vi "User Command Registers.vi"(0 "register instruction":T2) -> (4 "read completion":T1, 8 "IO Module\\User Command Idle":bool, 10 "IO Module\\User Error":u8, 14 "ready for input":bool)   [LabVIEW 2013]
uses:
  <instrlib>/ni579x/Register Bus/v1/FPGA/Public/Register Instruction.ctl
  <instrlib>/ni579x/Register Bus/v1/FPGA/Public/Read Completion.ctl
  <instrlib>/ni579x/Config/v1/Shared/Types/ni579x Register Bus Subsystem ID.ctl
  <vilib>/rvi/eio/common/nirviEmuTemplateMethod_errors.vi
  <vilib>/eio/EIONode/EIONode.xnode
  <vilib>/rvi/DataTransferAndStorage/Container/XNode/niFpgaContainer.xnode
  <instrlib>/ni579x/Register Bus/v1/FPGA/ni579x Register Bus v1 FPGA.lvlib
  <vilib>/rvi/interface/RandomDataEmulation/nirviRandomDataFpgaReadWriteTemplate.vi
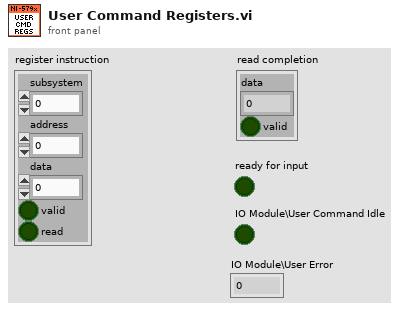
[diagram p1: front panel]
types:
  T1 = typedef "ni579x Register Bus v1 FPGA.lvlib/Read Completion.ctl" = cluster{"data":u32, "valid":bool}
  T2 = typedef "ni579x Register Bus v1 FPGA.lvlib/Register Instruction.ctl" = cluster{"subsystem":u8, "address":u16, "data":u32, "valid":bool, "read":bool}
  T3 = typedef "ni579x Register Bus Subsystem ID.ctl" = u8
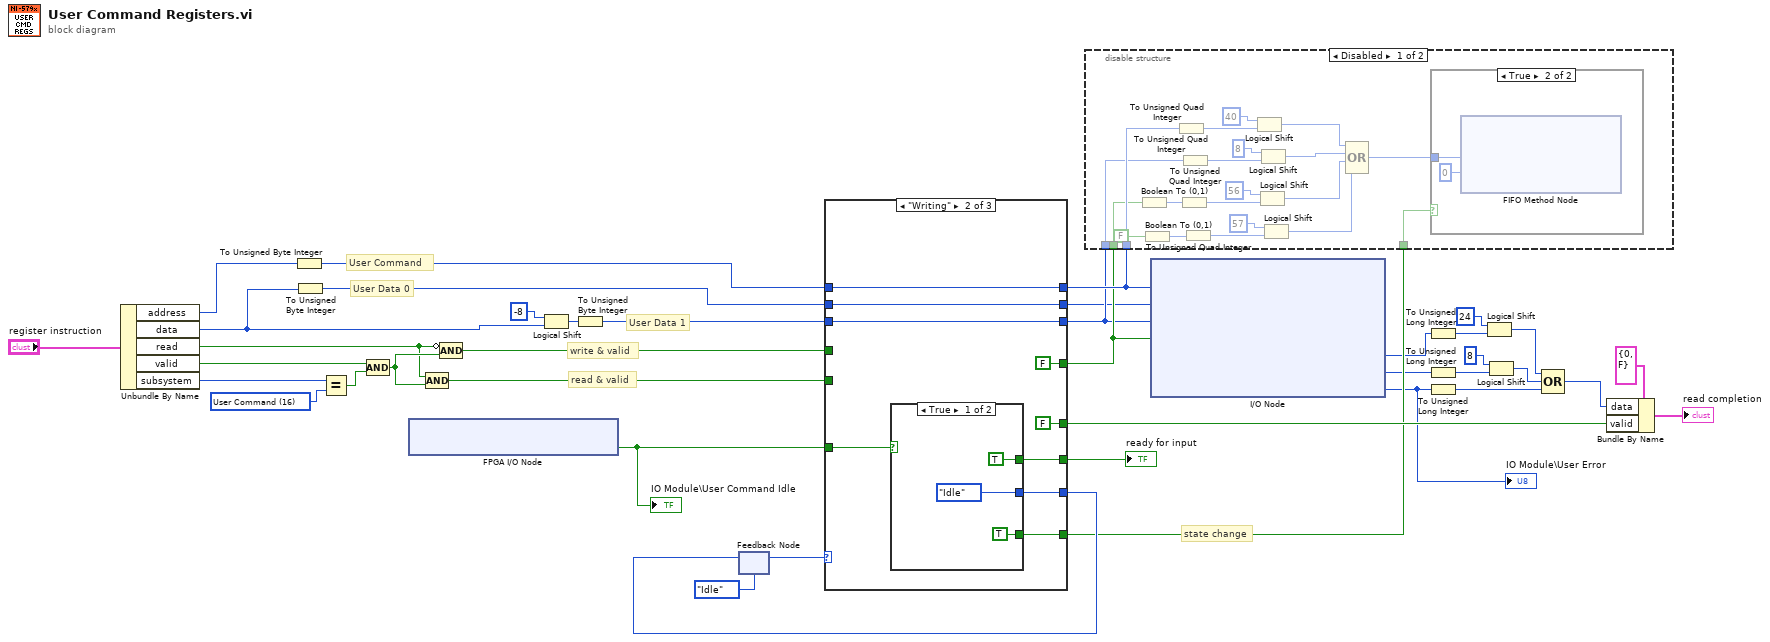
[diagram p0: block diagram]
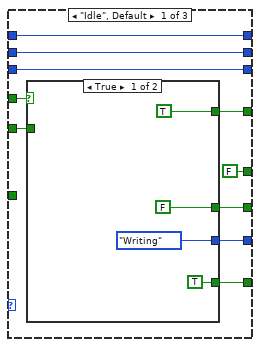
[diagram p4: hidden frame]
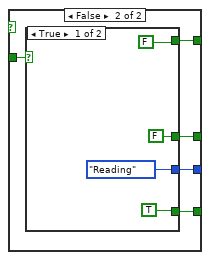
[diagram p5: hidden frame]
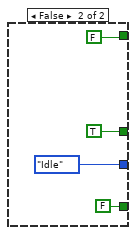
[diagram p6: hidden frame]
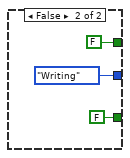
[diagram p7: hidden frame]
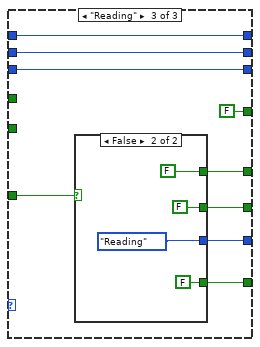
[diagram p8: hidden frame]
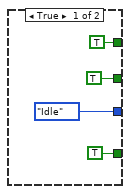
[diagram p9: hidden frame]
diagram:
  w2 = T3 16 items=["FAM Register Operation"=0, "User Command"=16, "Synchronization"=32] ("Subsystem ID")
  # "state change"
  # "User Command"
  # "User Data 1"
  # "User Data 0"
  # "read & valid"
  # "write & valid"
  n1 = Unbundle By Name("register instruction") -> ("address"=w27:u16, "data"=w3:u32, "read"=w37:bool, "valid"=w40:bool, "subsystem"=w1:u8)
  n2 = To Unsigned Byte Integer(number=w27) -> (unsigned 8bit integer=w26:u8)
  n3 = To Unsigned Byte Integer(number=w3) -> (unsigned 8bit integer=w22:u8)
  n4 = Equal?(x=w1, y=w2) -> (x = y?=w39:bool)
  n5 = Compound Arithmetic op=AND(w40, w39) -> (w38:bool)
  n6 = xnode "FPGA I/O Node"() -> ("IO Module\\User Command Idle"=w7:bool)  [unwired: 1 in, 1 out]
  "IO Module\\User Command Idle" <- w7
  n7 = Compound Arithmetic op=AND(w37, w38) -> (w33:bool)
  n8 = Compound Arithmetic op=AND(invert w37, w38) -> (w34:bool)
  n9 = Logical Shift(y=i16 -8, x=w3) -> (x << y=w23:u32)
  n10 = To Unsigned Byte Integer(number=w23) -> (unsigned 8bit integer=w21:u8)
  n11 = feedback #1(enum16{"Idle", "Writing", "Reading"}."Idle") -> (w35:enum16{"Idle", "Writing", "Reading"})
  n12 = case shown="\"Writing\"" w35 {
    tunnel: w26 -> [w49 w75 w90]
    tunnel: w21 -> [w48 w74 w89]
    tunnel: w34 -> [w50 _ _]
    tunnel: w33 -> [w46 _ _]
    tunnel: [w49 w75 w90] -> w30
    tunnel: [w48 w74 w89] -> w25
    tunnel: [w47 FALSE FALSE] -> w29
    tunnel: [w45 w71 w87] -> w32
    tunnel: [FALSE FALSE w85] -> w31
    tunnel: w7 -> [_ w72 w88]
    tunnel: [w44 w70 w86] -> w6
    tunnel: [w42 w69 w84] -> w28
    tunnel: w22 -> [w41 w68 w83]
    tunnel: [w41 w68 w83] -> w20
    frame "Idle", Default {
      n13 = case shown="True" w50 {
        tunnel: [TRUE w59] -> w47
        tunnel: w46 -> [_ w58]
        tunnel: [enum16{"Idle", "Writing", "Reading"}."Writing" w57] -> w45
        tunnel: [FALSE w56] -> w44
        tunnel: [TRUE w55] -> w42
        frame True {
        }
        frame False {
          n14 = case shown="True" w58 {
            tunnel: [FALSE FALSE] -> w59
            tunnel: [enum16{"Idle", "Writing", "Reading"}."Reading" enum16{"Idle", "Writing", "Reading"}."Idle"] -> w57
            tunnel: [FALSE TRUE] -> w56
            tunnel: [TRUE FALSE] -> w55
            frame True {
            }
            frame False {
            }
          }
        }
      }
    }
    frame "Writing" {
      n15 = case shown="True" w72 {
        tunnel: [enum16{"Idle", "Writing", "Reading"}."Idle" enum16{"Idle", "Writing", "Reading"}."Writing"] -> w71
        tunnel: [TRUE FALSE] -> w70
        tunnel: [TRUE FALSE] -> w69
        frame True {
        }
        frame False {
        }
      }
    }
    frame "Reading" {
      n16 = case shown="False" w88 {
        tunnel: [enum16{"Idle", "Writing", "Reading"}."Idle" enum16{"Idle", "Writing", "Reading"}."Reading"] -> w87
        tunnel: [TRUE FALSE] -> w86
        tunnel: [TRUE FALSE] -> w85
        tunnel: [TRUE FALSE] -> w84
        frame True {
        }
        frame False {
        }
      }
    }
  }
  "ready for input" <- w6
  n17 = feedback-in #1(w32) -> ()
  n18 = disable-structure shown="Disabled" {
    disable-tunnel: w30 -> [w111 _]
    disable-tunnel: w29 -> [w109 _]
    disable-tunnel: w28 -> [w102 _]
    disable-tunnel: w25 -> [w101 _]
    frame Disabled {
      n19 = Boolean To (0,1)(Boolean=w109) -> (0, 1=w110:i16)
      n20 = Boolean To (0,1)(Boolean=FALSE) -> (0, 1=w108:i16)
      n21 = To Unsigned Quad Integer(1:w111) -> (0:w119:u64)
      n22 = To Unsigned Quad Integer(1:w110) -> (0:w115:u64)
      n23 = To Unsigned Quad Integer(1:w101) -> (0:w116:u64)
      n24 = To Unsigned Quad Integer(1:w108) -> (0:w113:u64)
      n25 = Logical Shift(y=i8 40, x=w119) -> (x << y=w107:u64)
      n26 = Logical Shift(y=i8 56, x=w115) -> (x << y=w105:u64)
      n27 = Logical Shift(y=i8 8, x=w116) -> (x << y=w106:u64)
      n28 = Logical Shift(y=i8 57, x=w113) -> (x << y=w104:u64)
      n29 = Compound Arithmetic op=OR(w107, w106, w105, w104) -> (w103:u64)
      n30 = case shown="True" w102 {
        tunnel: w103 -> [_ w121]
        frame False {
        }
        frame True {
          n31 = xnode ("FIFO Method Node")("Element"=w121, "Timeout"=0) -> ()  [unwired: 1 in, 2 out]
        }
      }
    }
    frame Enabled {
    }
  }
  n32 = xnode "I/O Node"("IO Module\\User Command"=w30, "IO Module\\User Data 0"=w20, "IO Module\\User Data 1"=w25, "IO Module\\User Command Commit"=w29) -> ("IO Module\\User Command Status"=w15:u8, "IO Module\\User Return"=w16:u16, "IO Module\\User Error"=w13:u8)  [unwired: 7 in, 7 out]
  "IO Module\\User Error" <- w13
  n33 = To Unsigned Long Integer(number=w15) -> (unsigned 32bit integer=w19:u32)
  n34 = To Unsigned Long Integer(number=w16) -> (unsigned 32bit integer=w14:u32)
  n35 = To Unsigned Long Integer(number=w13) -> (unsigned 32bit integer=w10:u32)
  n36 = Logical Shift(y=i8 24, x=w19) -> (x << y=w12:u32)
  n37 = Logical Shift(y=i8 8, x=w14) -> (x << y=w11:u32)
  n38 = Compound Arithmetic op=OR(w12, w11, w10) -> (w9:u32)
  n39 = Bundle By Name(cluster=T1 {"data"=0, "valid"=FALSE} ("read completion"), "data"=w9, "valid"=w31) -> (→"read completion":T1)
